vi "GetSetTestClass.vi"(7 "Set":bool, 11 "Test.lvclass":refnum<class "Test.lvclass">) -> (3 "Test.lvclass":refnum<class "Test.lvclass">)   [LabVIEW 2014, in "Test.lvclass"]
uses:
  Test.lvclass
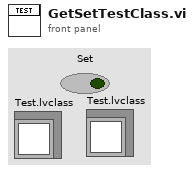
[diagram p1: front panel]
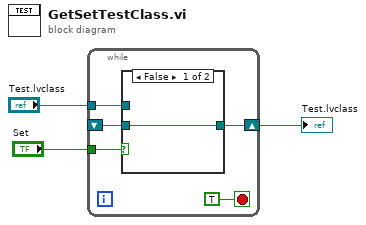
[diagram p0: block diagram]
diagram:
  n1 = while {
    shift-right: [w5] -> w1
    shift-left: _ -> [w4]
    tunnel: "Set" -> [w7]
    tunnel: "Test.lvclass" -> [w6]
    stop <- TRUE stop-if-true
    n2 = case shown="False" w7 {
      tunnel: w6 -> [_ w10]
      tunnel: [w9 w10] -> w5
      tunnel: w4 -> [w9 _]
      frame False {
      }
      frame True {
      }
    }
  }
  "Test.lvclass" <- w1
